vi "Read Data DVR.vi"(8 "error in (no error)":errorcluster, 11 "nCRD in":refnum<class "gCRD.lvclass">) -> (0 "error out":errorcluster, 2 "Data DVR":refnum<data-value>, 3 "nCRD out":refnum<class "gCRD.lvclass">)   [LabVIEW 2016, in "gCRDS.lvlib" / "gCRD.lvclass"]
uses:
  gCRD.lvclass
  Data/Nicholas Data.lvclass
  gCRD.lvclass/gCRD.ctl
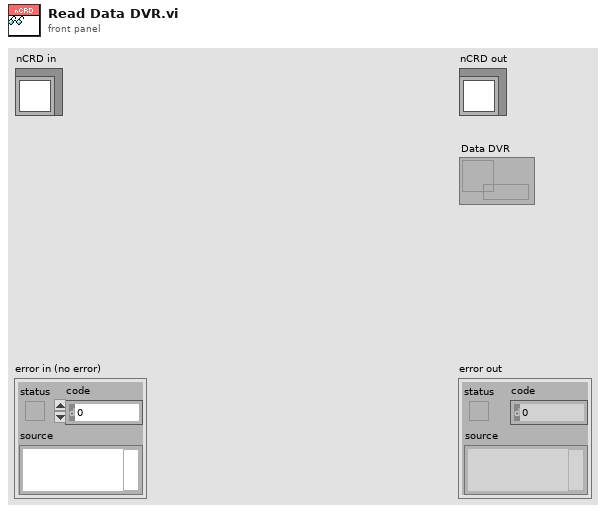
[diagram p1: front panel]
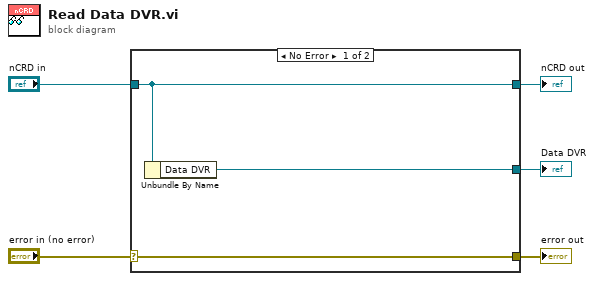
[diagram p0: block diagram]
diagram:
  n1 = case shown="No Error" "error in (no error)" {
    selector: "error in (no error)" -> [w8 w9]
    tunnel: [w8 w9] -> w4
    tunnel: [w7 w10] -> w2
    tunnel: "nCRD in" -> [w7 w10]
    tunnel: [w6 _] -> w1
    frame No Error {
      n2 = Unbundle By Name(w7) -> ("Data DVR"=w6:refnum<data-value>)
    }
    frame Error {
    }
  }
  "error out" <- w4
  "nCRD out" <- w2
  "Data DVR" <- w1
